vi "cRIO - Shared Variable RW.vi"(0 "shared variable RT Library":string="ni.var.psp://192.168.1.50/RT Library", 1 "Read/Write":T1=enum."Read", 3 "Data Path Name":string, 4 "cRIO Channel List (In)":i32[](array[numeric]), 5 "Error In":errorcluster, 6 "Simulate cRIO":bool, 7 "Probe List In":i32[](array[numeric]), 8 "cRIO Data Retention":i32, 10 "DAQ Start":bool, 12 "cRIO Status":refnum<vi>) -> (9 "cRIO Data Retention":i32, 11 "File IO Status":bool[](array[boolean]), 13 "Probe List Out":i32[](array[numeric]), 14 "data out":dbl[](array[numeric])=[28.24849025386229, 28.23947755526304, 28.19249680418221, 28.285480650091355, 1417.864336646555, 1417.864336646555, 1417.864336646555, 1417.864336646555], 15 "cRIO Timestamp":timestamp, 16 "Data Path Name":string, 17 "Cycle Count":i32, 18 "DAQ Started":bool, 19 "Error Out":errorcluster)   [LabVIEW 2013]
uses:
  Controls/cRIO RW Enum.ctl
panel:
  out "SV Close":errorcluster
  in  "Simulate DAQ Started":bool
  in  "subVI":bool=TRUE
  out "cRIO Status (internal)":string
  # "ni.var.psp://192.168.1.50/RT Library"
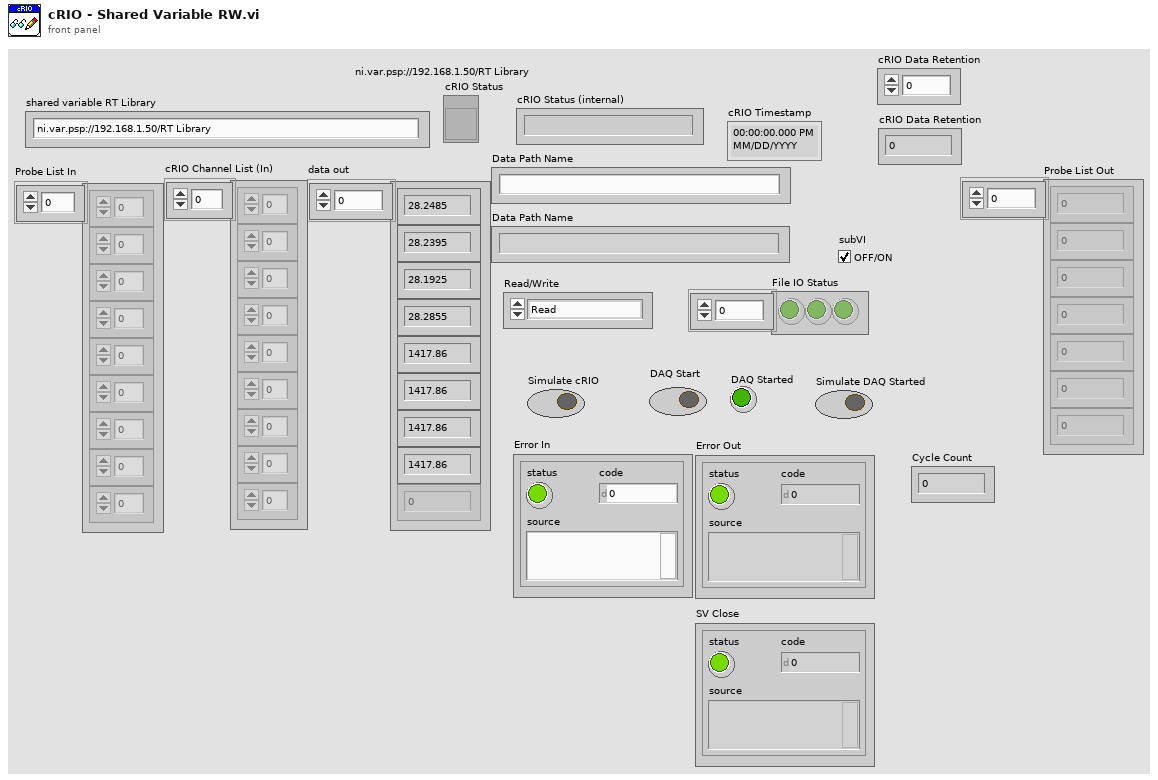
[diagram p1: front panel]
types:
  T1 = typedef "cRIO RW Enum.ctl" = enum16{"Write", "Read", "Write Others"}
  T2 = cluster{"Read Access":enum8{"Allowed", "Required", "None"}, "Write Access":enum8{"Allowed", "Required", "None"}}
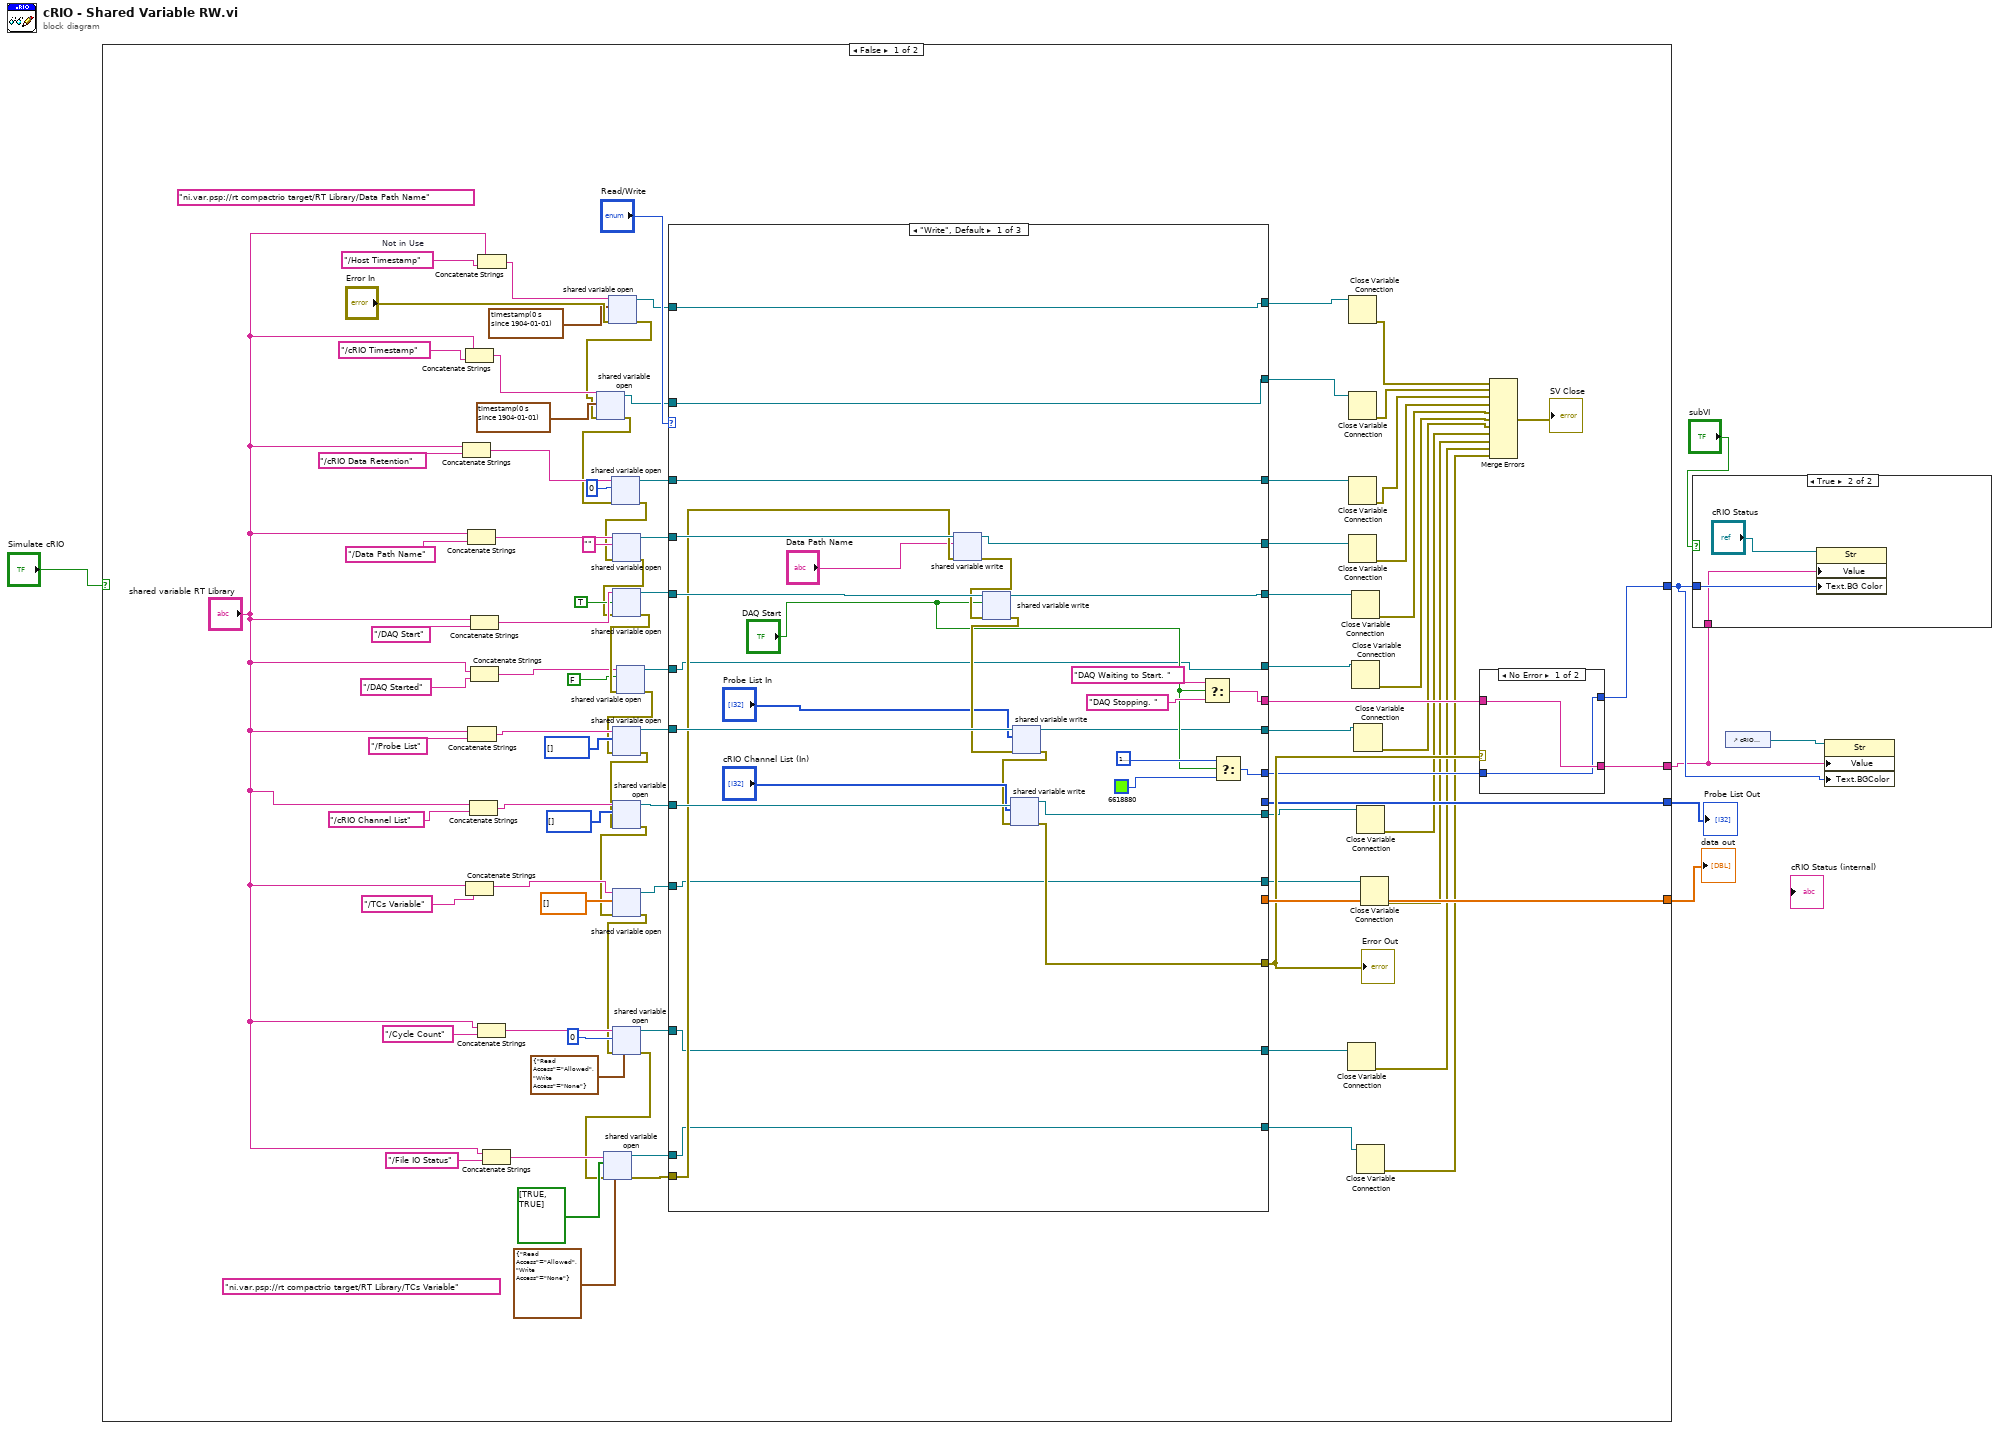
[diagram p0: block diagram]
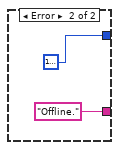
[diagram p3: hidden frame]
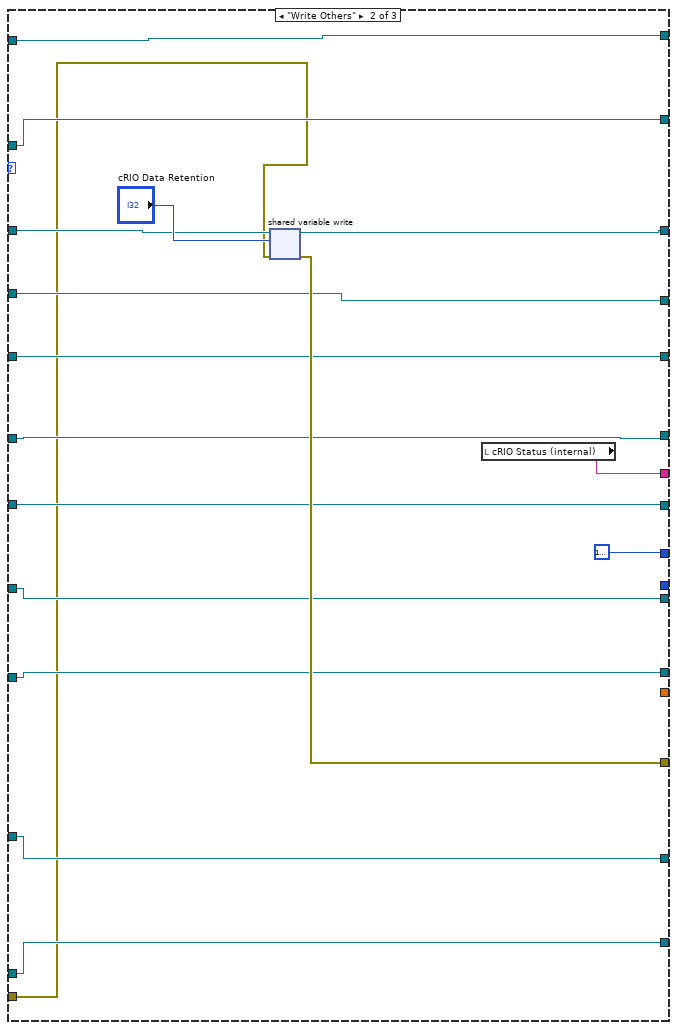
[diagram p4: hidden frame]
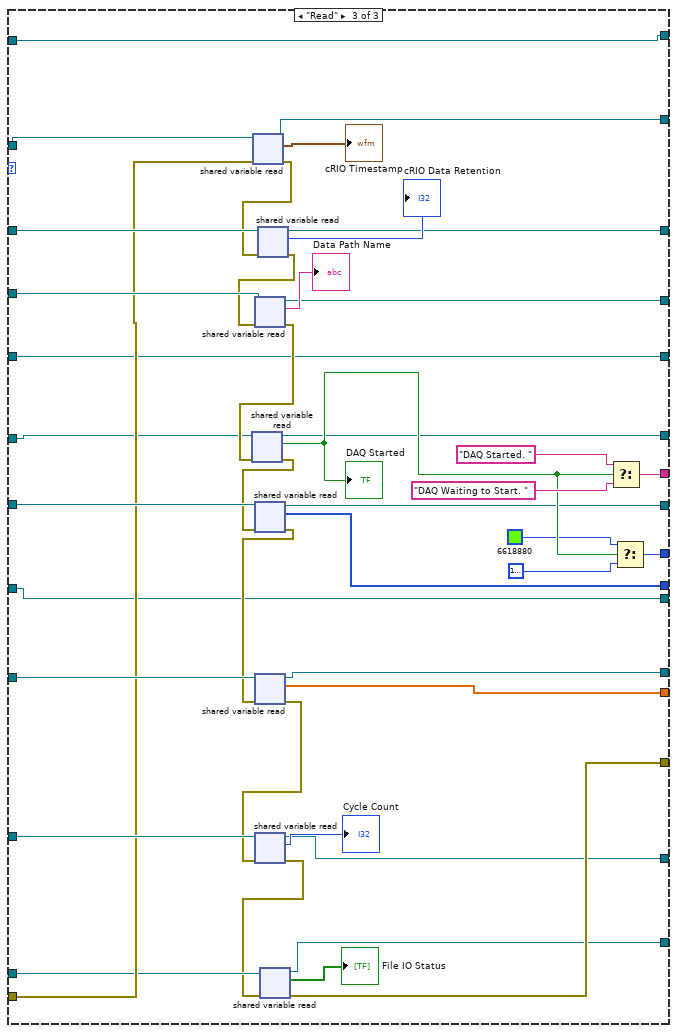
[diagram p5: hidden frame]
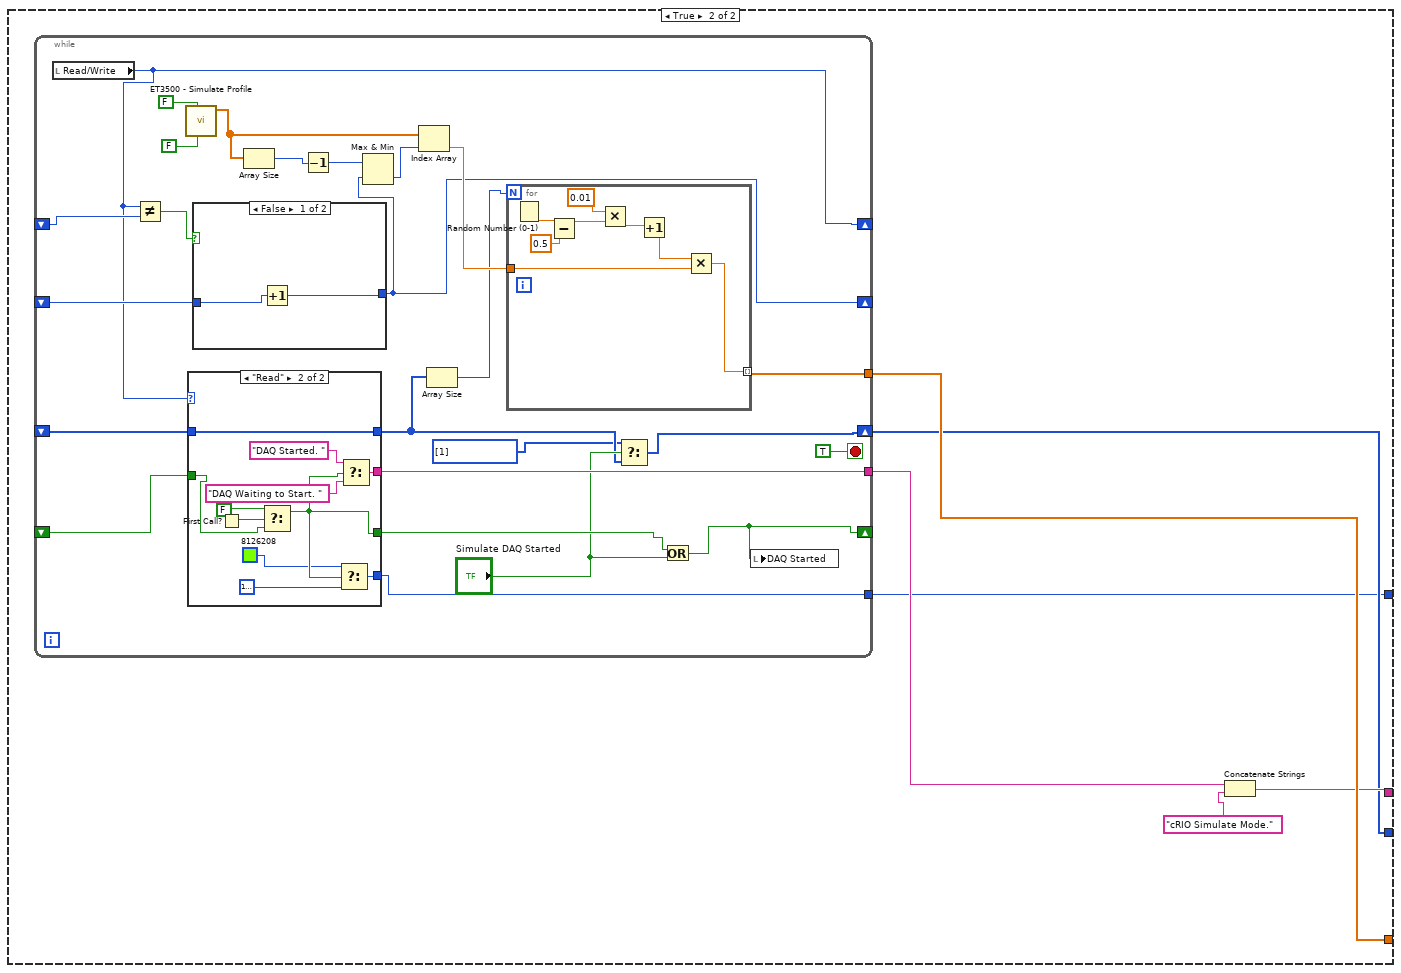
[diagram p6: hidden frame]
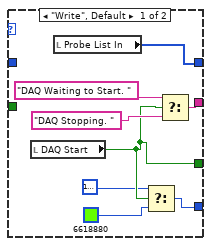
[diagram p7: hidden frame]
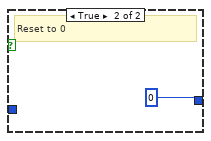
[diagram p8: hidden frame]
diagram:
  n1 = case shown="False" "Simulate cRIO" {
    tunnel: [w84 w196] -> w7
    tunnel: [w48 w194] -> w1
    tunnel: [w47 w192] -> w5
    tunnel: [w45 w191] -> w2
    frame False {
      w55 = "/Host Timestamp"  # Not in Use
      (unwired) "ni.var.psp://rt compactrio target/RT Library/Data Path Name"
      (unwired) "ni.var.psp://rt compactrio target/RT Library/TCs Variable"
      n2 = Concatenate Strings("shared variable RT Library", "/cRIO Data Retention" ("string")) -> (w64:string)
      n3 = Concatenate Strings("shared variable RT Library", "/cRIO Timestamp" ("string")) -> (w53:string)
      n4 = Concatenate Strings("shared variable RT Library", "/TCs Variable" ("string")) -> (w81:string)
      n5 = Concatenate Strings("shared variable RT Library", "/Data Path Name" ("string")) -> (w94:string)
      n6 = Concatenate Strings("shared variable RT Library", "/Probe List" ("string")) -> (w78:string)
      n7 = Concatenate Strings("shared variable RT Library", "/cRIO Channel List" ("string")) -> (w73:string)
      n8 = Concatenate Strings("shared variable RT Library", "/DAQ Start" ("string")) -> (w93:string)
      n9 = Concatenate Strings("shared variable RT Library", "/DAQ Started" ("string")) -> (w32:string)
      n10 = Concatenate Strings("shared variable RT Library", "/Cycle Count" ("string")) -> (w91:string)
      n11 = Concatenate Strings("shared variable RT Library", w55) -> (w56:string)
      n12 = Concatenate Strings("shared variable RT Library", "/File IO Status" ("string")) -> (w43:string)
      n13 = shared-variable-open(w56, "Error In", timestamp(0 s since 1904-01-01)) -> (w59:refnum<k21>, w51:errorcluster)  [unwired: 1 in]
      n14 = shared-variable-open(w53, w51, timestamp(0 s since 1904-01-01)) -> (w49:refnum<k21>, w50:errorcluster)  [unwired: 1 in]
      n15 = shared-variable-open(w64, w50, 0) -> (w61:refnum<k21>, w60:errorcluster)  [unwired: 1 in]
      n16 = shared-variable-open(w94, w60, "" ("string")) -> (w76:refnum<k21>, w69:errorcluster)  [unwired: 1 in]
      n17 = shared-variable-open(w93, w69, TRUE) -> (w87:refnum<k21>, w35:errorcluster)  [unwired: 1 in]
      n18 = shared-variable-open(w32, w35, FALSE) -> (w31:refnum<k21>, w34:errorcluster)  [unwired: 1 in]
      n19 = shared-variable-open(w78, w34, i32[] []) -> (w77:refnum<k21>, w68:errorcluster)  [unwired: 1 in]
      n20 = shared-variable-open(w73, w68, i32[] []) -> (w71:refnum<k21>, w67:errorcluster)  [unwired: 1 in]
      n21 = shared-variable-open(w81, w67, dbl[] []) -> (w82:refnum<k21>, w70:errorcluster)  [unwired: 1 in]
      n22 = shared-variable-open(w91, w70, 0, T2 {"Read Access"=enum."Allowed", "Write Access"=enum."None"} ("access")) -> (w80:refnum<k21>, w39:errorcluster)
      n23 = shared-variable-open(w43, w39, bool[] [TRUE, TRUE], T2 {"Read Access"=enum."Allowed", "Write Access"=enum."None"} ("access")) -> (w41:refnum<k21>, w38:errorcluster)
      n24 = case shown="\"Write\", Default" "Read/Write" {
        tunnel: w76 -> [w131 w141 w190]
        tunnel: w87 -> [w130 w140 w155]
        tunnel: [_ _ w188] -> w84
        tunnel: w82 -> [w104 w136 w187]
        tunnel: w80 -> [w103 w135 w186]
        tunnel: w38 -> [w119 w133 w171]
        tunnel: w77 -> [w129 w138 w184]
        tunnel: w71 -> [w128 w137 w152]
        tunnel: [w123 w145 w161] -> w66
        tunnel: [w120 w148 w177] -> w65
        tunnel: w61 -> [w110 w146 w176]
        tunnel: w59 -> [w112 w132 w159]
        tunnel: w49 -> [w111 w142 w173]
        tunnel: [_ _ w169] -> w47
        tunnel: [w115 u32 16777216 ("Color Box") w165] -> w46
        tunnel: w41 -> [w102 w134 w164]
        tunnel: w31 -> [w107 w139 w160]
        tunnel: [w112 w132 w159] -> w30
        tunnel: [w111 w142 w158] -> w29
        tunnel: [w110 w143 w156] -> w28
        tunnel: [w109 w141 w157] -> w27
        tunnel: [w108 w140 w155] -> w26
        tunnel: [w107 w139 w154] -> w25
        tunnel: [w106 w138 w153] -> w24
        tunnel: [w105 w137 w152] -> w23
        tunnel: [w104 w136 w151] -> w22
        tunnel: [w103 w135 w150] -> w21
        tunnel: [w102 w134 w149] -> w20
        frame "Write", Default {
          n25 = shared-variable-write(w131, w119, "Data Path Name") -> (w109:refnum<k21>, w126:errorcluster)
          n26 = shared-variable-write(w130, w126, "DAQ Start") -> (w108:refnum<k21>, w125:errorcluster)
          n27 = shared-variable-write(w129, w125, "Probe List In") -> (w106:refnum<k21>, w124:errorcluster)
          n28 = shared-variable-write(w128, w124, "cRIO Channel List (In)") -> (w105:refnum<k21>, w123:errorcluster)
          n29 = Select(t="DAQ Waiting to Start. " ("Parameter (Text)"), s="DAQ Start", f="DAQ Stopping. " ("Parameter (Text)")) -> (s? t:f=w120:string)
          n30 = Select(t=u32 16777216 ("Color Box"), s="DAQ Start", f=u32 6618880 ("Color Box")) -> (s? t:f=w115:u32)
        }
        frame "Write Others" {
          n31 = shared-variable-write(w146, w133, "cRIO Data Retention") -> (w143:refnum<k21>, w145:errorcluster)
          n32 = local read "cRIO Status (internal)"() -> (w148:string)
        }
        frame "Read" {
          n33 = shared-variable-read(w173, w171) -> (w158:refnum<k21>, w170:errorcluster, →"cRIO Timestamp":timestamp)  [unwired: 1 out]
          n34 = shared-variable-read(w176, w170) -> (w156:refnum<k21>, w175:errorcluster, →"cRIO Data Retention":i32)  [unwired: 1 out]
          n35 = shared-variable-read(w190, w175) -> (w157:refnum<k21>, w183:errorcluster, →"Data Path Name":string)  [unwired: 1 out]
          n36 = shared-variable-read(w160, w183) -> (w154:refnum<k21>, w182:errorcluster, w168:bool)  [unwired: 1 out]
          "DAQ Started" <- w168
          n37 = shared-variable-read(w184, w182) -> (w153:refnum<k21>, w181:errorcluster, w169:i32[])  [unwired: 1 out]
          n38 = shared-variable-read(w187, w181) -> (w151:refnum<k21>, w180:errorcluster, w188:dbl[])  [unwired: 1 out]
          n39 = shared-variable-read(w186, w180) -> (w150:refnum<k21>, w163:errorcluster, →"Cycle Count":i32)  [unwired: 1 out]
          n40 = shared-variable-read(w164, w163) -> (w149:refnum<k21>, w161:errorcluster, →"File IO Status":bool[])  [unwired: 1 out]
          n41 = Select(t="DAQ Started. " ("Parameter (Text)"), s=w168, f="DAQ Waiting to Start. " ("Parameter (Text)")) -> (s? t:f=w177:string)
          n42 = Select(t=u32 6618880 ("Color Box"), s=w168, f=u32 16777216 ("Color Box")) -> (s? t:f=w165:u32)
        }
      }
      "Error Out" <- w66
      n43 = Close Variable Connection(11:w21) -> (0:w10:errorcluster)  [unwired: 1 in]
      n44 = Close Variable Connection(11:w30) -> (0:w19:errorcluster)  [unwired: 1 in]
      n45 = Close Variable Connection(11:w29) -> (0:w18:errorcluster)  [unwired: 1 in]
      n46 = Close Variable Connection(11:w28) -> (0:w17:errorcluster)  [unwired: 1 in]
      n47 = Close Variable Connection(11:w27) -> (0:w16:errorcluster)  [unwired: 1 in]
      n48 = Close Variable Connection(11:w26) -> (0:w15:errorcluster)  [unwired: 1 in]
      n49 = Close Variable Connection(11:w25) -> (0:w14:errorcluster)  [unwired: 1 in]
      n50 = Close Variable Connection(11:w24) -> (0:w13:errorcluster)  [unwired: 1 in]
      n51 = Close Variable Connection(11:w23) -> (0:w12:errorcluster)  [unwired: 1 in]
      n52 = Close Variable Connection(11:w20) -> (0:w9:errorcluster)  [unwired: 1 in]
      n53 = Close Variable Connection(11:w22) -> (0:w11:errorcluster)  [unwired: 1 in]
      n54 = case shown="No Error" w66 {
        tunnel: [w99 "Offline." ("Parameter (Text)")] -> w48
        tunnel: w65 -> [w99 _]
        tunnel: w46 -> [w98 _]
        tunnel: [w98 u32 16777216 ("Color Box")] -> w45
        frame No Error {
        }
        frame Error {
        }
      }
      n55 = Merge Errors(w19, w18, w17, w16, w15, w14, w13, w12, w11, w10, w9) -> (→"SV Close":errorcluster)
    }
    frame True {
      n56 = while {
        tunnel: [w219] -> w196
        shift-right: [w208] -> _
        shift-left: _ -> [w216]
        shift-right: [w212] -> _
        shift-left: _ -> [w214]
        shift-right: [w197] -> w192
        shift-left: _ -> [w207]
        tunnel: [w206] -> w193
        shift-right: [w201] -> _
        shift-left: _ -> [w204]
        tunnel: [w203] -> w191
        stop <- TRUE stop-if-true
        n57 = local read "Read/Write"() -> (w208:T1)
        n58 = Not Equal?(x=w208, y=w216) -> (x != y?=w215:bool)
        n59 = call "ET3500 - Simulate Profile.vi"("Popup"=FALSE ("subVI"), "Set (T) / Get (F)"=FALSE) -> ("Data"=w213:dbl[])  [unwired: 5 in, 4 out]
        n60 = case shown="\"Read\"" w208 {
          tunnel: w207 -> [_ w240]
          tunnel: [w226 w240] -> w199
          tunnel: [w227 w237] -> w206
          tunnel: [w225 w233] -> w202
          tunnel: w204 -> [_ w234]
          tunnel: [w222 w230] -> w203
          frame "Write", Default {
            n61 = local read "DAQ Start"() -> (w225:bool)
            n62 = local read "Probe List In"() -> (w226:i32[])
            n63 = Select(t=u32 16777216 ("Color Box"), s=w225, f=u32 6618880 ("Color Box")) -> (s? t:f=w222:u32)
            n64 = Select(t="DAQ Waiting to Start. " ("Parameter (Text)"), s=w225, f="DAQ Stopping. " ("Parameter (Text)")) -> (s? t:f=w227:string)
          }
          frame "Read" {
            n65 = First Call?() -> (First Call?: T/F=w236:bool)
            n66 = Select(t=FALSE ("DAQ Start"), s=w236, f=w234) -> (s? t:f=w233:bool)
            n67 = Select(t=u32 8126208 ("Color Box"), s=w233, f=u32 16777216 ("Color Box")) -> (s? t:f=w230:u32)
            n68 = Select(t="DAQ Started. " ("Parameter (Text)"), s=w233, f="DAQ Waiting to Start. " ("Parameter (Text)")) -> (s? t:f=w237:string)
          }
        }
        n69 = case shown="False" w215 {
          tunnel: [w241 0] -> w212
          tunnel: w214 -> [w242 _]
          frame False {
            n70 = Increment(x=w242) -> (x+1=w241:i32)
          }
          frame True {
            # "Reset to 0"
          }
        }
        n71 = Array Size(array=w213) -> (size(s)=w211:i32)
        n72 = Decrement(x=w211) -> (x-1=w210:i32)
        n73 = Max & Min(x=w210, y=w212) -> (min(x,y)=w209:i32)  [unwired: 1 out]
        n74 = Index Array(array=w213, index=w209) -> (element=w220:dbl)
        n75 = Array Size(array=w199) -> (size(s)=w205:i32)
        n76 = for {
          N: w205 -> [_]
          tunnel: [w245] -> w219 mode=indexing
          tunnel: w220 -> [w246]
          n77 = Random Number (0-1)() -> (number: 0 to 1=w244:dbl)
          n78 = Subtract(x=w244, y=0.5) -> (x-y=w249:dbl)
          n79 = Multiply(x=0.01, y=w249) -> (x*y=w251:dbl)
          n80 = Increment(x=w251) -> (x+1=w247:dbl)
          n81 = Multiply(x=w247, y=w246) -> (x*y=w245:dbl)
        }
        n82 = Select(t=i32[] [1] ("Probe List In"), s="Simulate DAQ Started", f=w199) -> (s? t:f=w197:i32[])
        n83 = Or(x=w202, y="Simulate DAQ Started") -> (x .or. y?=w201:bool)
        n84 = local write "DAQ Started"(w201) -> ()
      }
      n85 = Concatenate Strings(w193, "cRIO Simulate Mode." ("Parameter (Text)")) -> (w194:string)
    }
  }
  "data out" <- w7
  "Probe List Out" <- w5
  n86 = case shown="True" "subVI" {
    tunnel: w2 -> [_ w253]
    tunnel: w1 -> [_ w252]
    frame False {
    }
    frame True {
      n87 = property class="Str"(reference="cRIO Status", "Value"=w252, "Text.BG Color"=w253) -> ()  [unwired: 1 in, 2 out]
    }
  }
  n88 = control-ref of="cRIO Status (internal)"() -> (w4:refnum<vi>)
  n89 = property class="Str"(reference=w4, "Value"=w1, "Text.BGColor"=w2) -> ()  [unwired: 1 in, 2 out]
